vi "DHE_SetAsyncExp.vi"(2 "DHE_asyncexp":bool) -> ()   [LabVIEW 2016]
uses:
  private/vis/DHE_VarAction.ctl
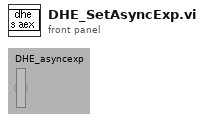
[diagram p1: front panel]
types:
  T1 = typedef "DHE_VarAction.ctl" = enum16{"read", "write"}
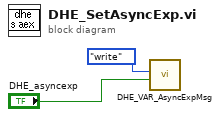
[diagram p0: block diagram]
diagram:
  n1 = call "DHE_VAR_AsyncExpMsg.vi"("value"="DHE_asyncexp", "action"=DHE_VarAction."write") -> ()  [unwired: 10 out]
